vi "getNumerator.vi"(8 "error in (no error)":errorcluster, 11 "IRatio in":refnum<class "IRatio.lvclass">) -> (0 "error out":errorcluster, 2 "Numerator out":i64, 3 "IRatio out":refnum<class "IRatio.lvclass">)   [LabVIEW 2022 SP3, in "openDAQ.lvlib" / "daqCoreTypes.lvlib" / "IRatio.lvclass"]
uses:
  <instrlib>/openDAQ/Public/Classes/daqCoreTypes/IRatio/IRatio.lvclass
  C:/Program Files (x86)/National Instruments/LabVIEW 2022/instr.lib/openDAQ/Public/Classes/IBaseObject/IBaseObject.lvclass
  <instrlib>/openDAQ/Public/Classes/IBaseObject/IBaseObject.lvclass/IBaseObject.ctl
  <instrlib>/openDAQ/Public/Classes/IBaseObject/Accessor/Read reference.vi
  <instrlib>/openDAQ/Binaries/Windows/x86/copendaq32.dll
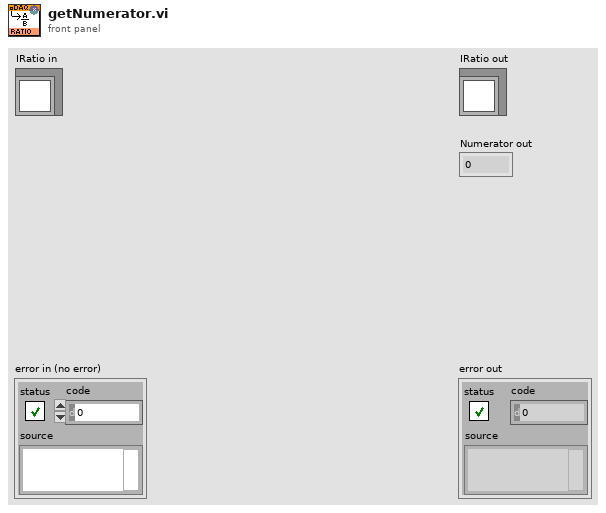
[diagram p1: front panel]
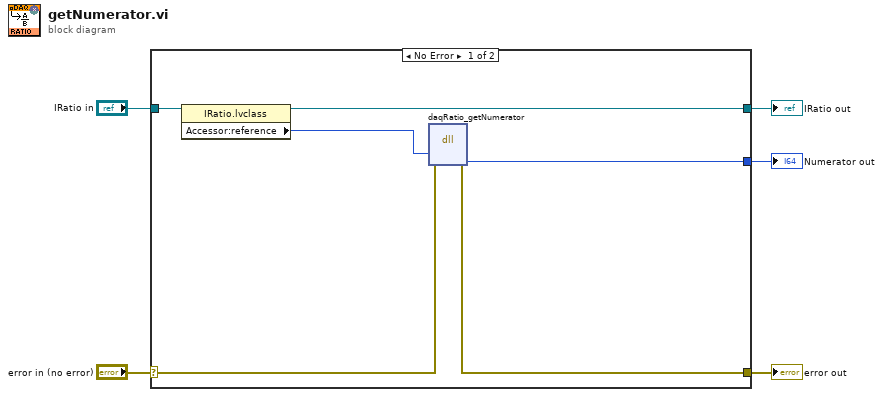
[diagram p0: block diagram]
diagram:
  n1 = case shown="No Error" "error in (no error)" {
    selector: "error in (no error)" -> [w10 w13]
    tunnel: [w9 w13] -> w4
    tunnel: [w6 w12] -> w3
    tunnel: "IRatio in" -> [w11 w12]
    tunnel: [w7 _] -> w2
    frame No Error {
      n2 = property class="IRatio.lvclass"(reference=w11) -> (reference out=w6:refnum<class "IRatio.lvclass">, "Accessor:reference"=w8:i64)  [unwired: 1 in, 1 out]
      n3 = dll-call lib="C:/Program Files (x86)/National Instruments/LabVIEW 2022/instr.lib/openDAQ/Binaries/Windows/x86/copendaq*.*" fn="daqRatio_getNumerator"(error in=w10, "ratio"=w8) -> (error out=w9:errorcluster, "numerator"=w7:i64)  [unwired: 5 in, 1 out]
    }
    frame Error {
    }
  }
  "error out" <- w4
  "IRatio out" <- w3
  "Numerator out" <- w2
